vi "Reorder Functions on Priority.vi"(0 "config path":path, 5 "Function List":string[](array[string]), 11 "error in (no error)":errorcluster) -> (6 "Function List out":string[](array[string]), 15 "error out":errorcluster)   [LabVIEW 2016, in "scripts manager.lvclass"]
uses:
  scripts manager.lvclass
  <vilib>/Utility/config.llb/Read Key (Boolean).vi
  <vilib>/Utility/config.llb/NI_LVConfig.lvlib
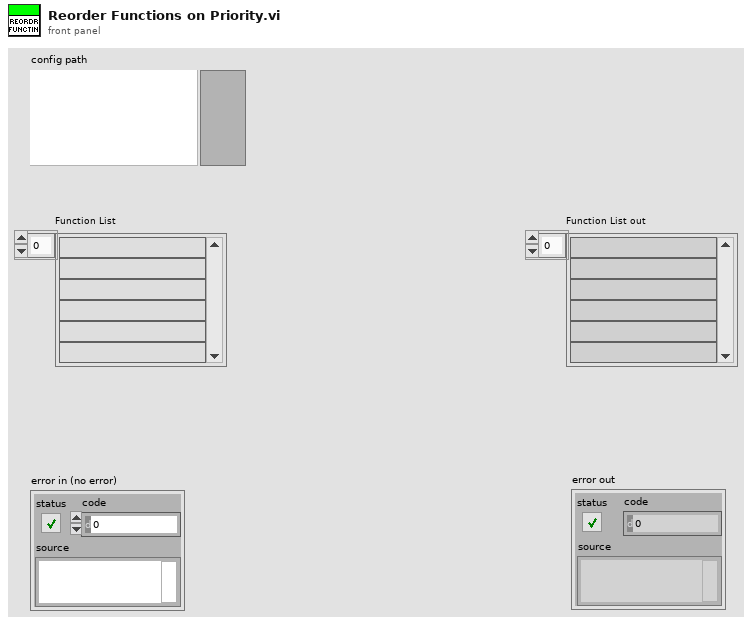
[diagram p1: front panel]
types:
  T1 = typedef "NI_LVConfig.lvlib/Config Data RefNum.ctl" = refnum<k1>
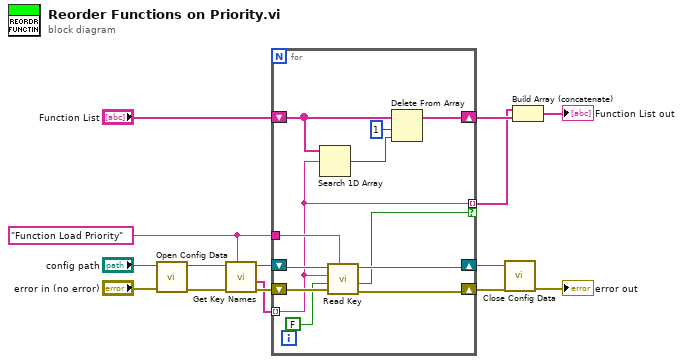
[diagram p0: block diagram]
diagram:
  w8 = "Function Load Priority" ("section")
  n1 = call <vilib>:"Open Config Data.vi"("error in (no error)"="error in (no error)", "configuration file path"="config path") -> ("error out"=w12:errorcluster, "refnum"=w13:T1)  [unwired: 7 in, 1 out]
  n2 = call <vilib>:"Get Key Names.vi"("section"=w8, "error in (no error)"=w12, "refnum"=w13) -> ("error out"=w11:errorcluster, "key names"=w9:string[], "refnum out"=w10:T1)  [unwired: 5 in, 1 out]
  n3 = for {
    shift-right: [w23] -> w6
    shift-left: w10 -> [w27]
    shift-right: [w24] -> w7
    shift-left: w11 -> [w26]
    tunnel: w9 -> [w17] mode=indexing
    tunnel: w8 -> [w22]
    shift-right: [w20] -> w3
    shift-left: "Function List" -> [w21]
    tunnel: [w17] -> w2 mode=indexing if=w16
    n4 = Search 1D Array(1D array=w21, element=w17) -> (index of element=w19:i32)  [unwired: 1 in]
    n5 = call-poly <vilib>:"Read Key.vi"("section"=w22, "error in (no error)"=w26, "default value"=FALSE, "key"=w17, "refnum"=w27) -> ("error out"=w24:errorcluster, "value"=w16:bool, "refnum out"=w23:T1)  [unwired: 3 in, 1 out]
    n6 = Delete From Array(array=w21, length=1, index=w19) -> (array with subset deleted=w20:string[])  [unwired: 1 out]
  }
  n7 = call <vilib>:"Close Config Data.vi"("error in (no error)"=w7, "refnum"=w6) -> ("error out"=→"error out":errorcluster)  [unwired: 8 in, 1 out]
  n8 = Build Array (concatenate)(w2, w3) -> (→"Function List out":string[])
